vi "poll.vi"(8 "error in (no error)":errorcluster, 11 "input_poller in":refnum<class "input_poller.lvclass">) -> (0 "error out":errorcluster, 3 "input_poller out":refnum<class "input_poller.lvclass">)   [LabVIEW 2015, in "input_poller.lvclass"]
uses:
  input_poller.lvclass
  input_poller.lvclass/input_poller.ctl
  <vilib>/ActorFramework/Actor/Actor.lvclass/Actor.ctl
  <vilib>/ActorFramework/Message Enqueuer/Message Enqueuer.lvclass/Message Enqueuer.ctl
  <vilib>/ActorFramework/Message Enqueuer/Enqueue.vi
  <vilib>/ActorFramework/Message Enqueuer/Init from Existing Queue.vi
  <vilib>/ActorFramework/Message Priority Queue/Priority Enqueue.vi
  <vilib>/ActorFramework/Stop Msg/Stop Msg.lvclass
  <vilib>/ActorFramework/Message Enqueuer/Message Enqueuer.lvclass
  <vilib>/ActorFramework/Actor/Actor.lvclass
  Result/Result.lvclass
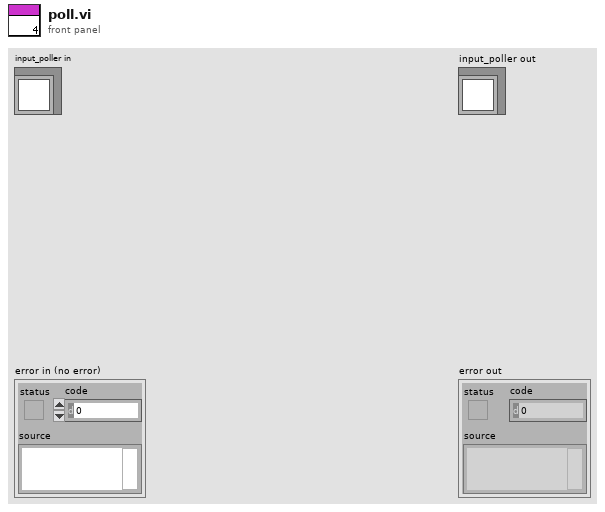
[diagram p1: front panel]
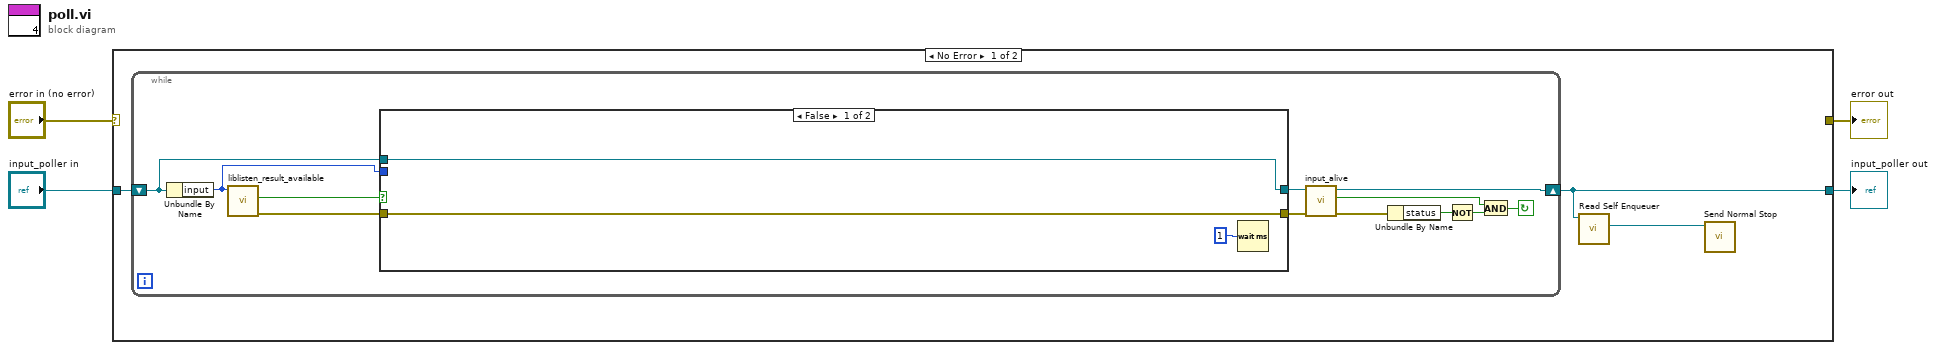
[diagram p0: block diagram]
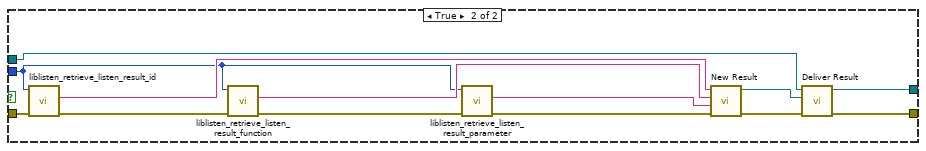
[diagram p2: hidden frame]
diagram:
  n1 = case shown="No Error" "error in (no error)" {
    selector: "error in (no error)" -> [_ w37]
    tunnel: [_ w37] -> w1
    tunnel: [w5 w36] -> w2
    tunnel: "input_poller in" -> [w7 w36]
    frame No Error {
      n2 = while {
        shift-right: [w19] -> w5
        shift-left: w7 -> [w13]
        stop <- w8 continue-if-true
        n3 = Unbundle By Name(w13) -> ("input"=w14:i32)
        n4 = call "liblisten_result_available.vi"("input"=w14) -> ("error out"=w17:errorcluster, "is"=w18:bool)  [unwired: 9 in]
        n5 = case shown="False" w18 {
          tunnel: w17 -> [w22 w35]
          tunnel: [w22 w25] -> w16
          tunnel: [w21 w26] -> w15
          tunnel: w14 -> [_ w24]
          tunnel: w13 -> [w21 w23]
          frame False {
            n6 = Wait (ms)(milliseconds to wait=u32 1) -> ()  [unwired: 1 out]
          }
          frame True {
            n7 = call "liblisten_retrieve_listen_result_id.vi"("error in (no error)"=w35, "input"=w24) -> ("error out"=w34:errorcluster, "id"=w32:string)  [unwired: 8 in]
            n8 = call "liblisten_retrieve_listen_result_function.vi"("error in (no error)"=w34, "input"=w24) -> ("error out"=w33:errorcluster, "function"=w31:string)  [unwired: 8 in]
            n9 = call "liblisten_retrieve_listen_result_parameter.vi"("error in (no error)"=w33, "input"=w24) -> ("error out"=w29:errorcluster, "parameter"=w30:string)  [unwired: 8 in]
            n10 = call "New Result.vi"("error in (no error)"=w29, "parameter"=w30, "function"=w31, "id"=w32) -> ("error out"=w28:errorcluster, "result"=w27:refnum<class "Result.lvclass">)  [unwired: 6 in]
            n11 = call-dynamic "Deliver Result.vi"("error in (no error)"=w28, "result"=w27, "input_poller in"=w23) -> ("error out"=w25:errorcluster, "input_poller out"=w26:refnum<class "input_poller.lvclass">)  [unwired: 7 in]
          }
        }
        n12 = call "input_alive.vi"("error in (no error)"=w16, "input_poller in"=w15) -> ("error out"=w12:errorcluster, "alive"=w9:bool, "input_poller out"=w19:refnum<class "input_poller.lvclass">)  [unwired: 7 in]
        n13 = Unbundle By Name(w12) -> ("status"=w11:bool)
        n14 = Not(x=w11) -> (.not. x?=w10:bool)
        n15 = And(x=w9, y=w10) -> (x .and. y?=w8:bool)
      }
      n16 = call <vilib>:"Read Self Enqueuer.vi"("Actor"=w5) -> ("Self Enqueuer"=w6:refnum<class "Message Enqueuer.lvclass">)  [unwired: 10 in]
      n17 = call <vilib>:"Send Normal Stop.vi"("Message Enqueuer"=w6) -> ()  [unwired: 10 in, 1 out]
    }
    frame Error {
    }
  }
  "error out" <- w1
  "input_poller out" <- w2
